vi "UpdateSingleParameter.vi"(1 "Value":string="aUI", 2 "Parameter":string="CameraAttributes::AcquisitionControl::AcquisitionFrameRate = \"", 3 "Camera config in":string) -> (0 "Camera config out":string)   [LabVIEW 2021]
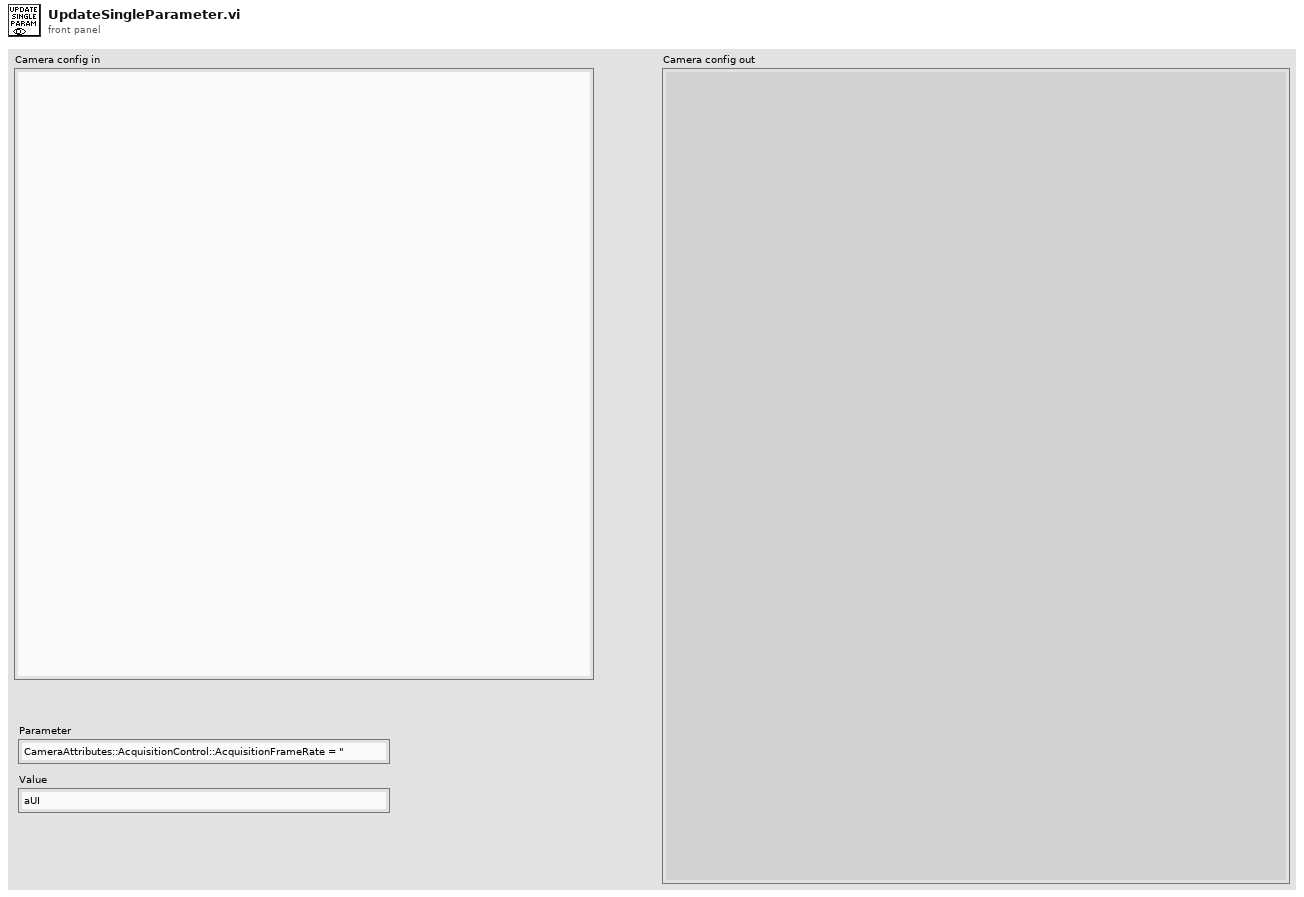
[diagram p1: front panel]
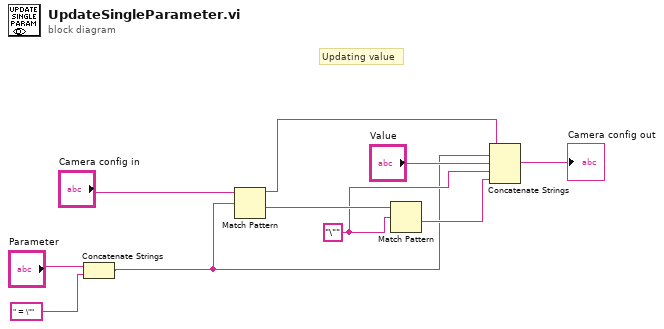
[diagram p0: block diagram]
diagram:
  w7 = "\"" ("regular expression")
  # "Updating value"
  n1 = Concatenate Strings("Parameter", " = \"") -> (w2:string)
  n2 = Match Pattern(string="Camera config in", regular expression=w2) -> (before substring=w9:string, after substring=w10:string)  [unwired: 1 in, 2 out]
  n3 = Match Pattern(string=w10, regular expression=w7) -> (after substring=w6:string)  [unwired: 1 in, 3 out]
  n4 = Concatenate Strings(w9, w2, "Value", w7, w6) -> (→"Camera config out":string)
